vi "NTJ_OldVer_NT Write Number_Fast.vi"(7 "IsFast":bool, 8 "error in":errorcluster, 9 "Numeric":dbl, 11 "Name":string="Numeric") -> (0 "error out":errorcluster)   [LabVIEW 2019]
doc: "Write the double precision numeric to the named entry."
uses:
  <vilib>/Rock Robotics/Network Tables/Field Data.ctl
  <vilib>/Rock Robotics/Network Tables/Field Type.ctl
  <vilib>/Rock Robotics/Network Tables/Sequence.ctl
  <vilib>/Rock Robotics/Network Tables/Create Actual Table Name.vi
  From_NTJ/NTJ_Convert NT Boolean to LV String.vi
  From_NTJ/NTJ_Convert String to NT Boolean Array Buffer.vi
  From_NTJ/NTJ_Convert String to NT Numeric Array Buffer.vi
  From_NTJ/NTJ_Convert String to NT String Array Buffer.vi
  <vilib>/Rock Robotics/Network Tables/Convert NT Types.vi
  From_NTJ/NTJ_Build NT Field ID Buffer.vi
  <vilib>/Utility/error.llb/Clear Errors.vi
  <vilib>/Rock Robotics/Network Tables/NT Globals.vi
  <vilib>/Rock Robotics/Network Tables/Table Manager.vi
  <vilib>/Rock Robotics/Network Tables/Log Issues.vi
  From_NTJ/NTJ_Convert String to NT String Buffer.vi
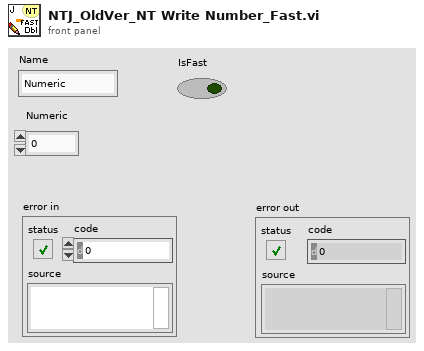
[diagram p1: front panel]
types:
  T1 = typedef "Field Data.ctl" = cluster{"Dbl":dbl, "String":string, "Type":T2, "Boolean":bool, "Sequence #":T3, "Flags":u8}
  T2 = typedef "Field Type.ctl" = enum8{"Invalid", "Bool", "Numeric", "String", "Raw", "Boolean Array", "Numeric Array", "String Array", "RPC"}
  T3 = typedef "Sequence.ctl" = u16
  T4 = enum16{"Update Field", "Read Field", "Assign Field", "Remove All", "Set Persistence", "Clear Persistence", "UpdValueLocal", "UpdValueServer", "UpdValueClient", "UpdFlags"}
  T5 = enum16{"Add Cnx", "Remove Cnx", "Retrieve List", "Cnx Inited"}
  T6 = typedef "Field ID.ctl" = i32
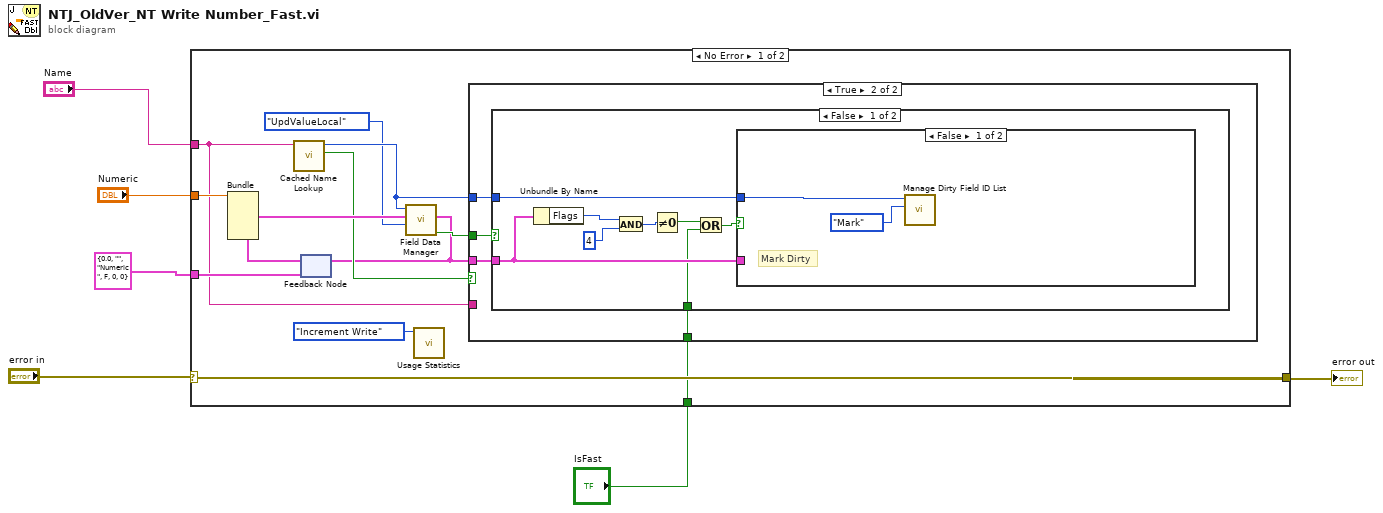
[diagram p0: block diagram]
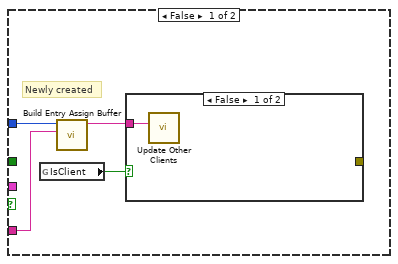
[diagram p2: hidden frame]
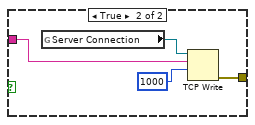
[diagram p3: hidden frame]
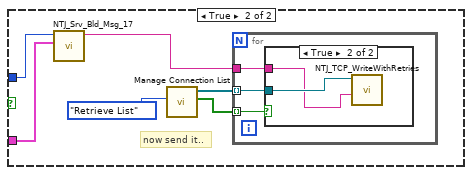
[diagram p4: hidden frame]
diagram:
  n1 = case shown="No Error" "error in" {
    selector: "error in" -> [w16 w54]
    tunnel: "Numeric" -> [w19 _]
    tunnel: "Name" -> [w11 _]
    tunnel: T1 {"Dbl"=0.0, "String"="", "Type"=enum."Numeric", "Boolean"=FALSE, "Sequence #"=0, "Flags"=0} ("Field Value In") -> [w18 _]
    tunnel: [w16 w54] -> w2
    tunnel: "IsFast" -> [w7 _]
    frame No Error {
      n2 = call <vilib>:"Cached Name Lookup.vi"("Name"=w11) -> ("Success"=w10:bool, "Entry ID"=w13:T6)  [unwired: 8 in, 1 out]
      n3 = feedback #1(w18) -> (w17:T1)
      n4 = Bundle(cluster=w17, "Dbl"=w19) -> (w12:T1)  [unwired: 5 in]
      n5 = call <vilib>:"Field Data Manager.vi"("Operation"=T4."UpdValueLocal", "Field Value In"=w12, "Field ID"=w13) -> ("Equal"=w15:bool, "Field Value Out"=w8:T1)  [unwired: 7 in]
      n6 = feedback-in #1(w8) -> ()
      n7 = call <vilib>:"Usage Statistics.vi"("Operation"=enum16{"Increment Read", "Increment Write"}."Increment Write") -> ()  [unwired: 11 in]
      n8 = case shown="True" w10 {
        tunnel: w13 -> [w23 w32]
        tunnel: w15 -> [_ w31]
        tunnel: w11 -> [w20 _]
        tunnel: w8 -> [_ w30]
        tunnel: w7 -> [_ w29]
        frame False {
          # "Newly created"
          n9 = global read "NT Globals.vi" "IsClient"() -> (w22:bool)
          n10 = call <vilib>:"Build Entry Assign Buffer.vi"("Name"=w20, "Field ID"=w23) -> ("data string"=w21:string)  [unwired: 9 in]
          n11 = case shown="False" w22 {
            tunnel: w21 -> [w24 w27]
            tunnel: [_ w25] -> _
            frame False {
              n12 = call <vilib>:"Update Other Clients.vi"("data string"=w24) -> ()  [unwired: 11 in]
            }
            frame True {
              n13 = global read "NT Globals.vi" "Server Connection"() -> (w28:refnum<k5>)
              n14 = TCP Write(connection ID=w28, data in=w27, 9:1000 ("timeout ms (25000)")) -> (error out=w25:errorcluster)  [unwired: 1 in, 2 out]
            }
          }
        }
        frame True {
          n15 = case shown="False" w31 {
            tunnel: w32 -> [w40 _]
            tunnel: w30 -> [w36 _]
            tunnel: w29 -> [w33 _]
            frame False {
              n16 = Unbundle By Name(w36) -> ("Flags"=w38:u8)
              n17 = And(x=w38, y=u8 4) -> (x .and. y?=w39:u8)
              n18 = Not Equal To 0?(x=w39) -> (x != 0?=w34:bool)
              n19 = Or(x=w34, y=w33) -> (x .or. y?=w35:bool)
              n20 = case shown="False" w35 {
                tunnel: w40 -> [w41 w48]
                tunnel: w36 -> [_ w47]
                frame False {
                  # "Mark Dirty"
                  n21 = call <vilib>:"Manage Dirty Field ID List.vi"("Operation"=enum16{"Mark", "Retrieve/Clear"}."Mark", "Field ID"=w41) -> ()  [unwired: 8 in, 2 out]
                }
                frame True {
                  # "now send it.."
                  n22 = call "NTJ_Srv_Bld_Msg_17.vi"("Field Value"=w47, "Field ID"=w48) -> ("Msg Buffer"=w43:string)  [unwired: 9 in]
                  n23 = call <vilib>:"Manage Connection List.vi"("Operation"=T5."Retrieve List") -> ("Inited"=w46:bool[], "Connections List"=w45:refnum<k5>[])  [unwired: 8 in, 1 out]
                  n24 = for {
                    tunnel: w45 -> [w50] mode=indexing
                    tunnel: w46 -> [w51] mode=indexing
                    tunnel: w43 -> [w49]
                    n25 = case shown="True" w51 {
                      tunnel: w50 -> [_ w53]
                      tunnel: w49 -> [_ w52]
                      frame False {
                      }
                      frame True {
                        n26 = call "NTJ_TCP_WriteWithRetries.vi"("Msg Buffer"=w52, "TCP Network Connection in"=w53) -> ()  [unwired: 8 in, 2 out]
                      }
                    }
                  }
                }
              }
            }
            frame True {
            }
          }
        }
      }
    }
    frame Error {
    }
  }
  "error out" <- w2
